vi "testSetFilter.vi"(8 "error in (no error)":errorcluster) -> (0 "error out":errorcluster)   [LabVIEW 2016]
doc: "Test the set/getFilter.vi."
uses:
  ZTAAC/ZTAAC.lvclass
  StrictDef/FilterType.ctl
  <vilib>/addons/_JKI Toolkits/Caraya/classes/Test/Test.lvclass
  OfcFunc.lvlib
  <vilib>/addons/_JKI Toolkits/Caraya/classes/Assert/Assert.lvclass
panel:
  in  "ZTAAC.lvclass":refnum<class "ZTAAC.lvclass">
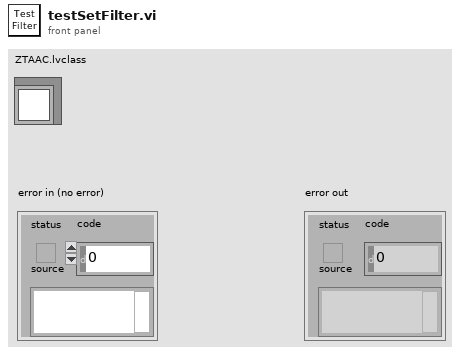
[diagram p1: front panel]
types:
  T1 = typedef "OfcFunc.lvlib/FilterType.ctl" = enum16{"ref", "u", "g", "r", "i", "z", "y"}
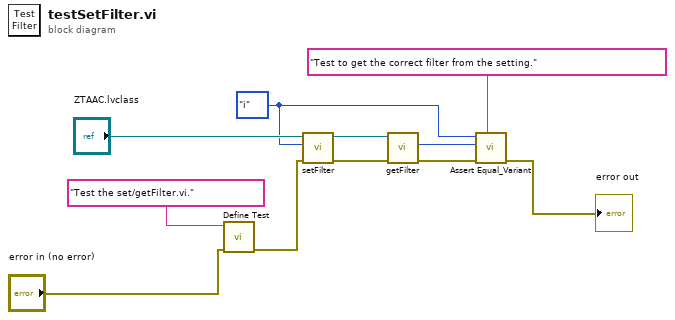
[diagram p0: block diagram]
diagram:
  w1 = FilterType."i" ("Filter Type")
  n1 = call <vilib>:"Define Test.vi"("error in (no error)"="error in (no error)", "Label (VI Title)"="Test the set/getFilter.vi.") -> ("error out"=w8:errorcluster)  [unwired: 9 in]
  n2 = call "setFilter.vi"("error in (no error)"=w8, "Filter Type"=w1, "ZTAAC in"="ZTAAC.lvclass") -> ("error out"=w6:errorcluster, "ZTAAC out"=w7:refnum<class "ZTAAC.lvclass">)  [unwired: 7 in]
  n3 = call "getFilter.vi"("error in (no error)"=w6, "ZTAAC in"=w7) -> ("error out"=w4:errorcluster, "Filter Type"=w5:T1)  [unwired: 7 in, 1 out]
  n4 = call <vilib>:"Assert Equal_Variant.vi"("Label"="Test to get the correct filter from the setting." ("Label (VI Title)"), "error in (no error)"=w4, "Y"=w5, "X"=w1) -> ("error out"=→"error out":errorcluster)  [unwired: 7 in]
